vi "configureB.vi"(0 "boolean array":bool[](array[boolean]), 1 "boolean":bool, 3 "Inkscape Offset":cluster{"X Offset":dbl, "Y Offset":dbl}, 4 "Inkscape Scaling":T2={"X Scaling (%)"=100.0, "Y Scaling (%)"=100.0}, 5 "string array":string[](array[string]), 6 "Rotation(degree)":dbl, 7 "shape properties":T1(array[cluster]), 8 "Canvas Size":cluster{"Width":dbl, "Height":dbl}={"Width"=35.0, "Height"=35.0}, 9 "order array reference":refnum<vi>, 10 "reset boolean reference":refnum<vi>) -> (2 "lithography data":T1(array[cluster]))   [LabVIEW 2013]
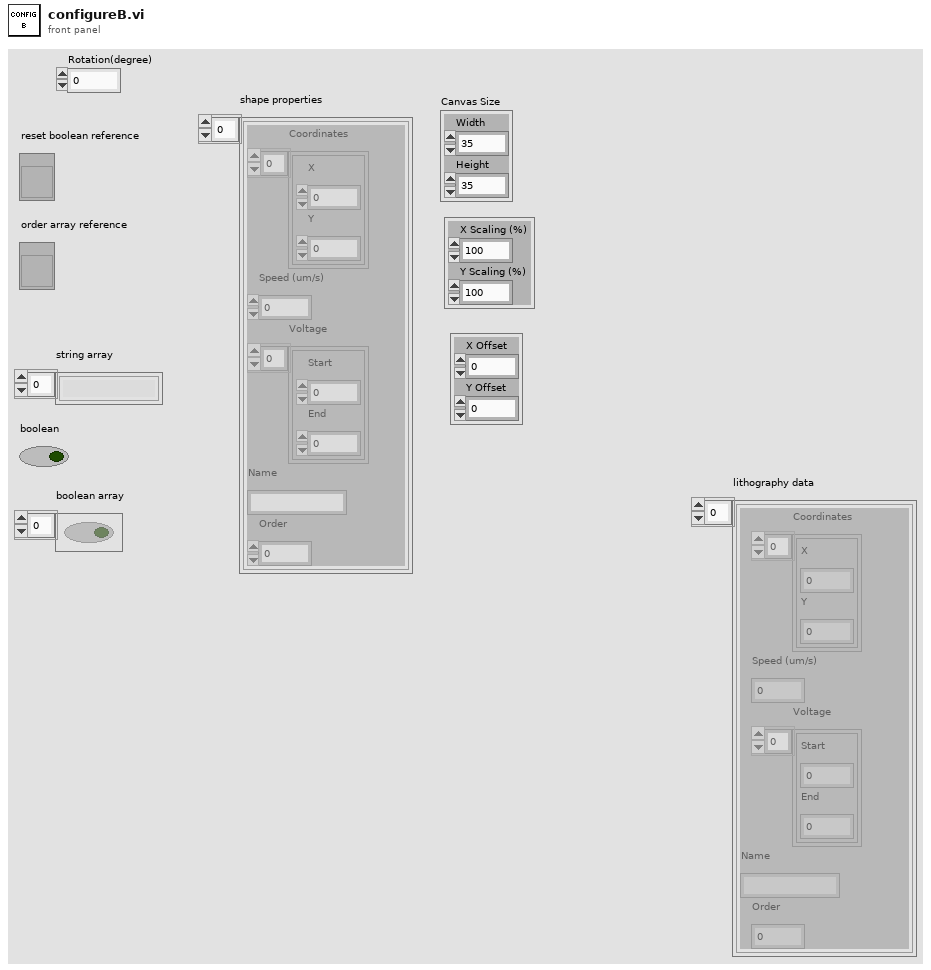
[diagram p1: front panel]
types:
  T1 = cluster{"Coordinates":cluster{"X":dbl, "Y":dbl}[], "Speed (um/s)":dbl, "Voltage":cluster{"Start":dbl, "End":dbl}[], "Name":string, "Order":i32}[]
  T2 = cluster{"X Scaling (%)":dbl, "Y Scaling (%)":dbl}
  T3 = cluster{"Name":string, bool, "Start Voltage":dbl, "Start Voltage":dbl}
  T4 = cluster{"Coordinates":cluster{"X":dbl, "Y":dbl}[], "Speed (um/s)":dbl, "Voltage":cluster{"Start":dbl, "End":dbl}[], "Name":string, "Order":i32}
  T5 = cluster{"String":string, "Boolean":bool, "Start Voltage":dbl, "Speed":dbl}[]
  T6 = cluster{"String":string, "Boolean":bool, "Start Voltage":dbl, "Speed":dbl}
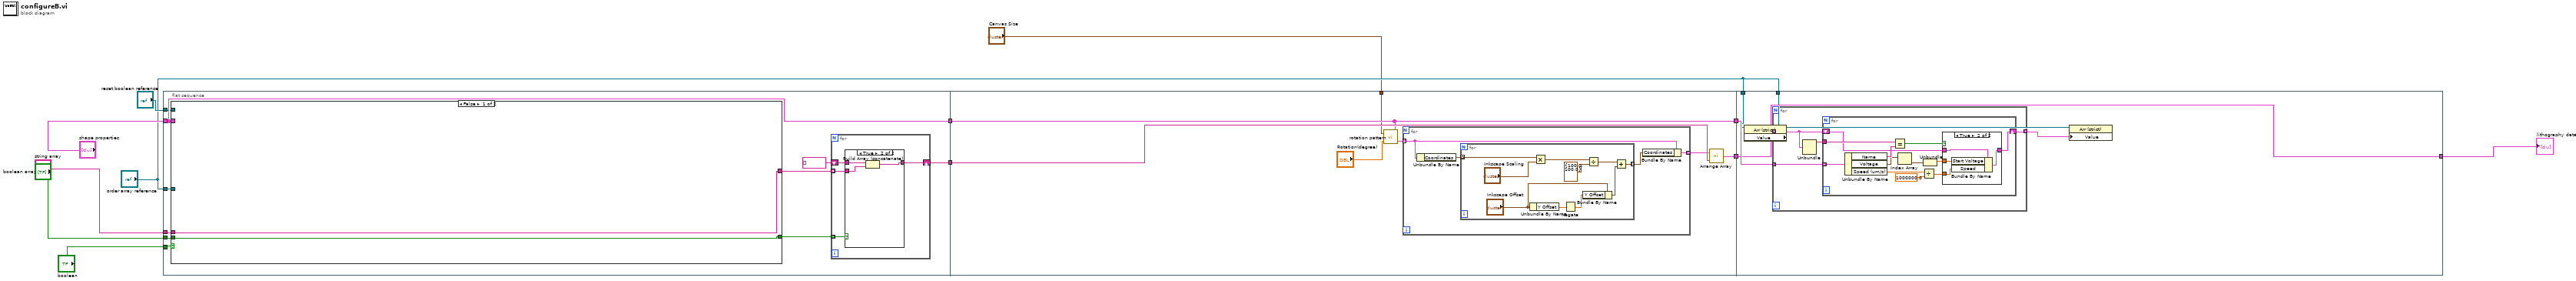
[diagram p0: block diagram]
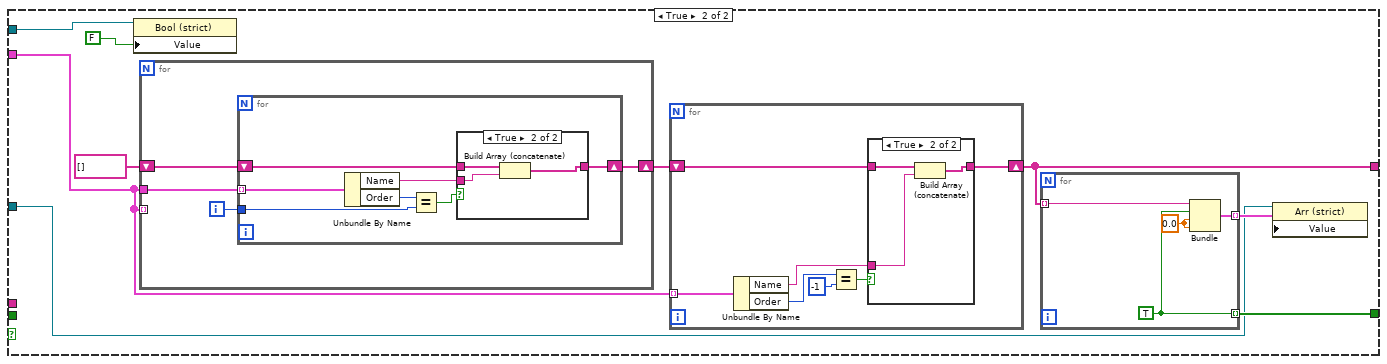
[diagram p2: hidden frame]
diagram:
  n1 = flat-sequence {
    tunnel: "shape properties" -> [w22]
    tunnel: [w22] -> w12
    tunnel: "string array" -> [w21]
    tunnel: "boolean array" -> [w18]
    tunnel: "boolean" -> [w15]
    tunnel: [w19] -> w11
    tunnel: "order array reference" -> [w14]
    tunnel: "reset boolean reference" -> [w13]
    tunnel: w12 -> [w76]
    tunnel: [w76] -> w10
    tunnel: [w77] -> w9
    tunnel: w11 -> [w78]
    tunnel: "Canvas Size" -> [w72]
    tunnel: w10 -> [w96]
    tunnel: [w95] -> w4
    tunnel: w9 -> [w95]
    tunnel: "order array reference" -> [w94]
    tunnel: "order array reference" -> [w93]
    frame #0 {
      n2 = case shown="False" w15 {
        tunnel: w22 -> [_ w29]
        tunnel: [w24 w28] -> w20
        tunnel: w21 -> [w24 _]
        tunnel: w18 -> [w23 _]
        tunnel: [w23 w33] -> w17
        tunnel: w14 -> [_ w26]
        tunnel: w13 -> [_ w25]
        frame False {
        }
        frame True {
          n3 = property class="Bool (strict)"(reference=w25, "Value"=FALSE ("Reset")) -> ()  [unwired: 1 in, 2 out]
          n4 = for {
            tunnel: w29 -> [w48]
            shift-right: [w47] -> w30
            shift-left: string[] [] -> [w45]
            tunnel: w29 -> [_] mode=indexing
            i -> [w46]
            n5 = for {
              tunnel: w48 -> [w55] mode=indexing
              tunnel: w46 -> [w53]
              shift-right: [w50] -> w47
              shift-left: w45 -> [w49]
              n6 = Unbundle By Name(w55) -> ("Name"=w51:string, "Order"=w54:i32)
              n7 = Equal?(x=w54, y=w53) -> (x = y?=w52:bool)
              n8 = case shown="True" w52 {
                tunnel: w51 -> [_ w59]
                tunnel: [w56 w58] -> w50
                tunnel: w49 -> [w56 w57]
                frame False {
                }
                frame True {
                  n9 = Build Array (concatenate)(w57, w59) -> (w58:string[])
                }
              }
            }
          }
          n10 = for {
            tunnel: w29 -> [w40] mode=indexing
            shift-right: [w36] -> w28
            shift-left: w30 -> [w35]
            n11 = Unbundle By Name(w40) -> ("Name"=w37:string, "Order"=w39:i32)
            n12 = Equal?(x=w39, y=-1) -> (x = y?=w38:bool)
            n13 = case shown="True" w38 {
              tunnel: w37 -> [_ w44]
              tunnel: [w41 w43] -> w36
              tunnel: w35 -> [w41 w42]
              frame False {
              }
              frame True {
                n14 = Build Array (concatenate)(w42, w44) -> (w43:string[])
              }
            }
          }
          n15 = for {
            tunnel: w28 -> [w63] mode=indexing
            tunnel: [w62] -> w33 mode=indexing
            tunnel: [w61] -> w27 mode=indexing
            w60 = 0.0 ("Start Voltage")
            w62 = TRUE
            n16 = Bundle("Name"=w63, w62, "Start Voltage"=w60, "Start Voltage"=w60) -> (w61:T3)  [unwired: 1 in]
          }
          n17 = property class="Arr (strict)"(reference=w26, "Value"=w27) -> ()  [unwired: 1 in, 2 out]
        }
      }
      n18 = for {
        tunnel: w20 -> [w67] mode=indexing
        tunnel: w17 -> [w64] mode=indexing
        shift-right: [w66] -> w19
        shift-left: string[] [] -> [w65]
        n19 = case shown="True" w64 {
          tunnel: w67 -> [_ w71]
          tunnel: [w68 w70] -> w66
          tunnel: w65 -> [w68 w69]
          frame False {
          }
          frame True {
            n20 = Build Array (concatenate)(w69, w71) -> (w70:string[])
          }
        }
      }
    }
    frame #1 {
      n21 = call "rotation pattern.vi"("Rotation array"=w76, "Rotation(degree)"="Rotation(degree)", "Inkscape Image Size"=w72) -> ("Rotated array"=w74:T1)
      n22 = for {
        tunnel: w74 -> [w81] mode=indexing
        tunnel: [w79] -> w73 mode=indexing
        n23 = Unbundle By Name(w81) -> ("Coordinates"=w82:cluster{"X":dbl, "Y":dbl}[])
        n24 = for {
          tunnel: [w89] -> w80 mode=indexing
          tunnel: w82 -> [w88] mode=indexing
          n25 = Unbundle By Name("Inkscape Offset") -> ("Y Offset"=w85:dbl)
          n26 = Multiply(x=w88, y="Inkscape Scaling") -> (x*y=w92:cluster{dbl, dbl})
          n27 = Negate(x=w85) -> (-x=w86:dbl)
          n28 = Bundle By Name(cluster="Inkscape Offset", "Y Offset"=w86) -> (w83:cluster{"X Offset":dbl, "Y Offset":dbl})
          n29 = Divide(x=w92, y=cluster{dbl, dbl} {100.0, 100.0}) -> (x/y=w90:cluster{dbl, dbl})
          n30 = Add(x=w90, y=w83) -> (x+y=w89:cluster{dbl, dbl})
        }
        n31 = Bundle By Name(cluster=w81, "Coordinates"=w80) -> (w79:T4)
      }
      n32 = call "Arrange Array.vi"("Order"=w78, "Arrange array"=w73) -> ("Arranged array"=w77:T1)
    }
    frame #2 {
      n33 = property class="Arr (strict)"(reference=w93) -> ("Value"=w98:T5)  [unwired: 1 in, 2 out]
      n34 = for {
        tunnel: w98 -> [w100] mode=indexing
        tunnel: [w101] -> w97 mode=indexing
        tunnel: w96 -> [w99]
        n35 = Unbundle(w100) -> ("String"=w102:string)  [unwired: 3 out]
        n36 = for {
          tunnel: w102 -> [w113]
          shift-right: [w111] -> w101
          shift-left: w100 -> [w110]
          tunnel: w99 -> [w109] mode=indexing
          n37 = Unbundle By Name(w109) -> ("Name"=w114:string, "Voltage"=w105:cluster{"Start":dbl, "End":dbl}[], "Speed (um/s)"=w108:dbl)
          n38 = Equal?(x=w113, y=w114) -> (x = y?=w112:bool)
          n39 = Index Array(array=w105) -> (element=w104:cluster{"Start":dbl, "End":dbl})  [unwired: 1 in]
          n40 = Divide(x=w108, y=1000000.0) -> (x/y=w106:dbl)
          n41 = Unbundle(w104) -> ("Start"=w103:dbl)  [unwired: 1 out]
          n42 = case shown="True" w112 {
            tunnel: w110 -> [w115 w119]
            tunnel: w103 -> [_ w118]
            tunnel: [w115 w117] -> w111
            tunnel: w106 -> [_ w116]
            frame False {
            }
            frame True {
              n43 = Bundle By Name(cluster=w119, "Start Voltage"=w118, "Speed"=w116) -> (w117:T6)
            }
          }
        }
      }
      n44 = property class="Arr (strict)"(reference=w94, "Value"=w97) -> ()  [unwired: 1 in, 2 out]
    }
  }
  "lithography data" <- w4
